vi "Test2.vi"() -> ()   [LabVIEW 2013]
panel:
  out "standard output 4":string
  out "standard error 4":string
  out "standard error 3":string
  out "standard output 3":string
  out "standard error 2":string
  out "standard output 2":string
  out "standard error":string
  out "return code":i32
  out "standard output":string
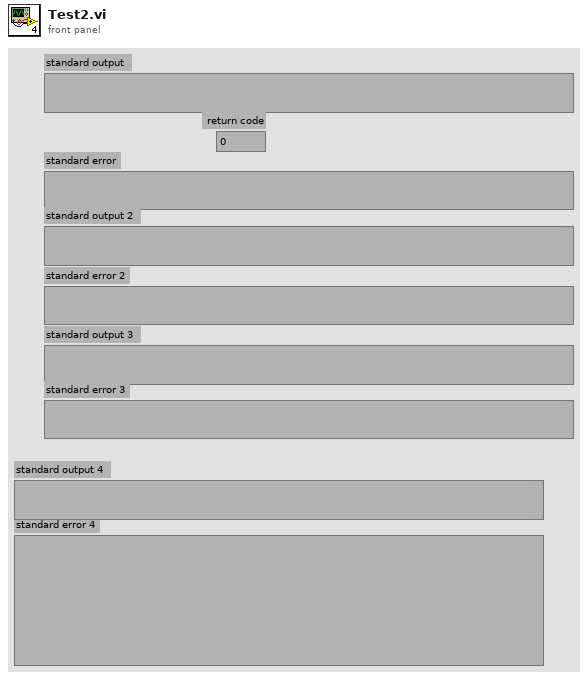
[diagram p1: front panel]
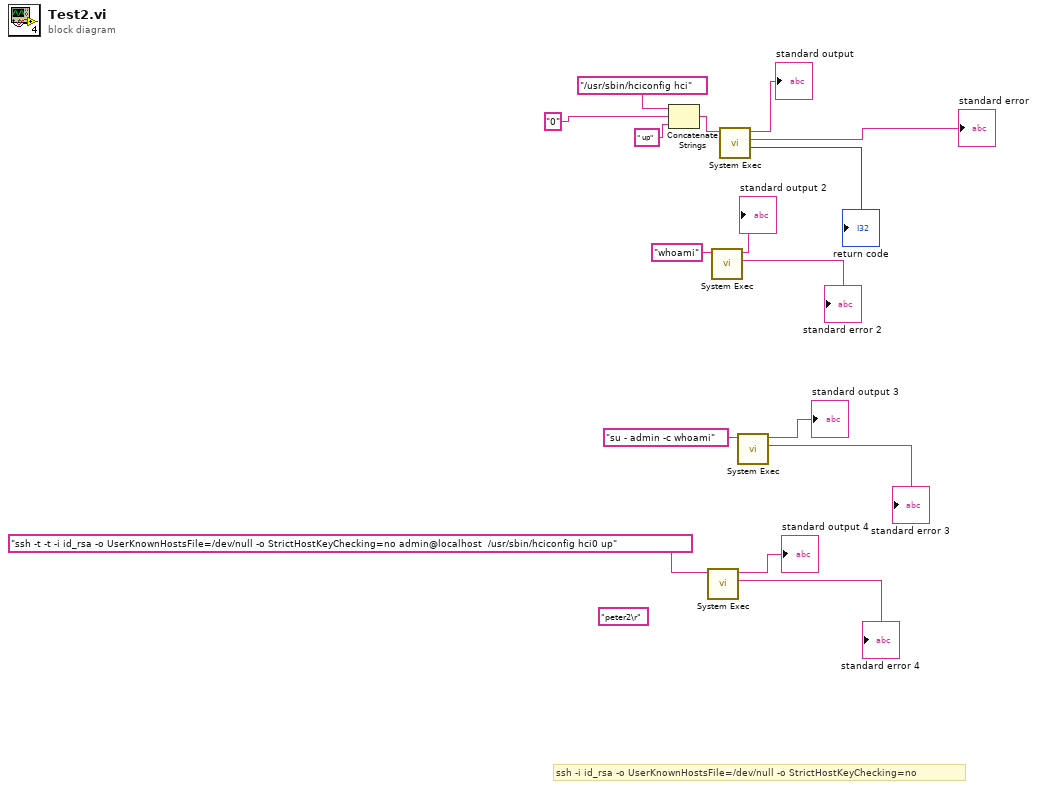
[diagram p0: block diagram]
diagram:
  (unwired) "peter2\r" ("standard input")
  # "ssh -i id_rsa -o UserKnownHostsFile=/dev/null -o StrictHostKeyChecking=no"
  n1 = Concatenate Strings("/usr/sbin/hciconfig hci" ("command line"), "0" ("string"), " up" ("string")) -> (w15:string)
  n2 = call <vilib>:"System Exec.vi"("command line"="ssh -t -t -i id_rsa -o UserKnownHostsFile=/dev/null -o StrictHostKeyChecking=no admin@localhost  /usr/sbin/hciconfig hci0 up") -> ("standard error"=→"standard error 4":string, "standard output"=→"standard output 4":string)  [unwired: 7 in, 2 out]
  n3 = call <vilib>:"System Exec.vi"("command line"="whoami") -> ("standard error"=→"standard error 2":string, "standard output"=→"standard output 2":string)  [unwired: 7 in, 2 out]
  n4 = call <vilib>:"System Exec.vi"("command line"=w15) -> ("return code"=→"return code":i32, "standard error"=→"standard error":string, "standard output"=→"standard output":string)  [unwired: 7 in, 1 out]
  n5 = call <vilib>:"System Exec.vi"("command line"="su - admin -c whoami") -> ("standard error"=→"standard error 3":string, "standard output"=→"standard output 3":string)  [unwired: 7 in, 2 out]
